vi "Read channels.vi"(8 "error in (no error)":errorcluster, 11 "Update Tag Config in":refnum<class "Update Tag Config.lvclass">) -> (0 "error out":errorcluster, 2 "Channels":refnum<class "TBM channel.lvclass">[](array[class]), 3 "Update Tag Config out":refnum<class "Update Tag Config.lvclass">)   [LabVIEW 2015, in "Update Tag Config.lvclass"]
uses:
  Update Tag Config.lvclass
  <vilib>/NI/Tag Bus Module Framework/channel/TBM channel.lvclass
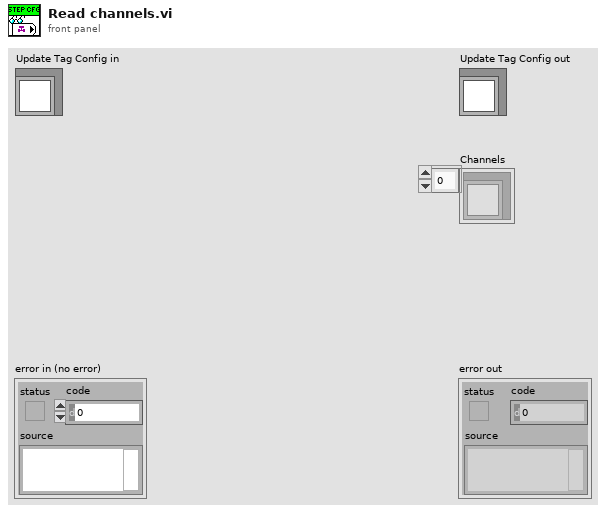
[diagram p1: front panel]
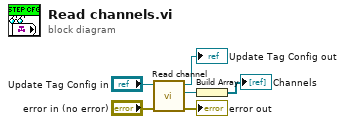
[diagram p0: block diagram]
diagram:
  n1 = call-dynamic "Read channel.vi"("error in (no error)"="error in (no error)", "Update Tag Config in"="Update Tag Config in") -> ("error out"=→"error out":errorcluster, "channel"=w4:refnum<class "TBM channel.lvclass">, "Update Tag Config out"=→"Update Tag Config out":refnum<class "Update Tag Config.lvclass">)  [unwired: 7 in]
  n2 = Build Array(w4) -> (→"Channels":refnum<class "TBM channel.lvclass">[])
